vi "TabControl-EnDis.vi"(8 "Error In":errorcluster, 9 "Tab":i32, 10 "Tab Enabled State":T1(ring), 11 "TabControl in":refnum<vi>) -> (0 "Error Out":errorcluster)   [LabVIEW 2021]
doc: "André Romero - 2021\nandretec@ifsc.usp.br"
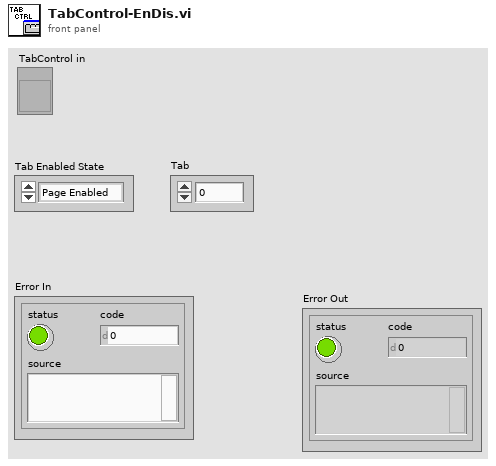
[diagram p1: front panel]
types:
  T1 = enum32{"Page Enabled", "Page Disabled", "Page Disabled & Grayed"}
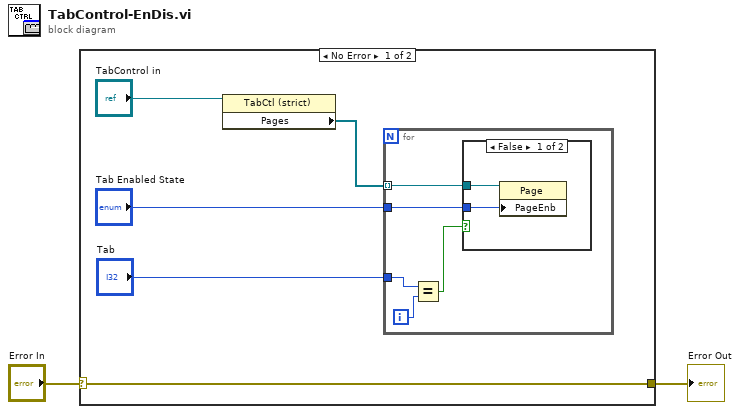
[diagram p0: block diagram]
diagram:
  n1 = case shown="No Error" "Error In" {
    selector: "Error In" -> [w6 w15]
    tunnel: [w6 w15] -> w1
    frame No Error {
      n2 = property on="Property Node" class="TabCtl (strict)"(reference="TabControl in") -> ("Pages"=w4:refnum<vi>[])  [unwired: 1 in, 2 out]
      n3 = for {
        tunnel: "Tab Enabled State" -> [w12]
        tunnel: w4 -> [w11] mode=indexing
        tunnel: "Tab" -> [w9]
        i -> [w10]
        n4 = Equal?(x=w9, y=w10) -> (x = y?=w8:bool)
        n5 = case shown="False" w8 {
          tunnel: w12 -> [w14 _]
          tunnel: w11 -> [w13 _]
          frame False {
            n6 = property class="Page"(reference=w13, "PageEnb"=w14) -> ()  [unwired: 1 in, 2 out]
          }
          frame True {
          }
        }
      }
    }
    frame Error {
    }
  }
  "Error Out" <- w1
